vi "SVXMPL_Initialize.vi"(0 "device":i16=1, 1 "acquisition type":T1(ring), 5 "output channels":tag[](array[tag]), 9 "input channels":tag[](array[tag]), 11 "error in (no error)":errorcluster) -> (4 "acquisition task":T2={"AI device settings"={"AI device"=1, "AI taskID"=0, "response"=[]}, "acquisition type"=enum."Finite", "measurement settings"={"AI sampling frequency"=51200.0, "AO sampling frequency"=51200.0, "AI block size"=1024, "AO block Size"=0, "block duration [ms]"=1024.0, "number of AI channels"=0, "board propagation time [samples]"=0, "DUT propagation time [s]"=0.0}, "settling settings"={"settle time"=0.015599999576807022, "settle cycles"=5}, "integration settings"={"integration time"=0.015599999576807022, "integration cycles"=5}, "AO device settings"={"AO device"=1, "AO taskID"=0, "excitation"=[]}, "acquisition accounting"={"initial read size [samples]"=0, "read offset [samples]"=0, "read length [samples]"=0, "blocks to settle [samples]"=0, "min delay until transition [samples]"=0}, "frequency range"={"start frequency"=0.015599999576807022, "stop frequency"=5.0}, "block type"=enum."Initialize", "source settings"={"signal type"=enum."Dual tone (IMD)", "frequency"=0.0, "total amplitude"=0.0, "frequencies"=[1.0], "relative amplitudes"=[1.0], "offset"=1.0, "total amplitude list"=[1.0], "ramping rate"=0.0}} {"source settings"."total amplitude" format="%.2f"; "source settings"."relative amplitudes" format="%.2f"; "source settings"."frequencies" format="%.2f"; "source settings"."total amplitude list" format="%.2f"; "source settings"."ramping rate" format="%.4f"; "source settings"."offset" format="%.2f"; "source settings"."frequency" format="%.2f"; "frequency range"."stop frequency" format="%.2f"; "frequency range"."start frequency" format="%.2f"; "AO device settings"."excitation"."output limits"."low limit (-10 V)" format="%.2f"; "AO device settings"."excitation"."output limits"."high limit (10 V)" format="%.2f"; "AI device settings"."response"."input limits"."low limit (0.0)" format="%.2f"; "AI device settings"."response"."input limits"."high limit (0.0)" format="%.2f"; "integration settings"."integration time" format="%.2p"; "settling settings"."settle time" format="%.2p"; "measurement settings"."DUT propagation time [s]" format="%.2f"; "measurement settings"."AO sampling frequency" format="%.2f"; "measurement settings"."AI sampling frequency" format="%.2f"}, 15 "error out":errorcluster)   [LabVIEW 2017]
doc: "This example VI allows you to configure the <B>device</B>, <B>output channel</B>, and <B>input channels</B> that will be used for the synchronized AO/AI measurement. The device must support both input and output to use this VI.\n\nYou must also specify the <B>aquisition type</B> that will be performed.\n\"Finite\" is a one-shot measurement.\n\"Averaged\" is a continuous measurement in which measured blocks are averaged.\n\"Settled\" is a continuous measurement in which measured blocks are tested against the settling criteria. If the measurement is settled, only the last measurement is returned.\n\"Amplitude sweep\" is a continuous measurement in which each measured block has a different amplitude for the test signal."
uses:
  <vilib>/addons/Sound and Vibration/compatibility/Example Support/SVXMPL_Acquisition Task.ctl
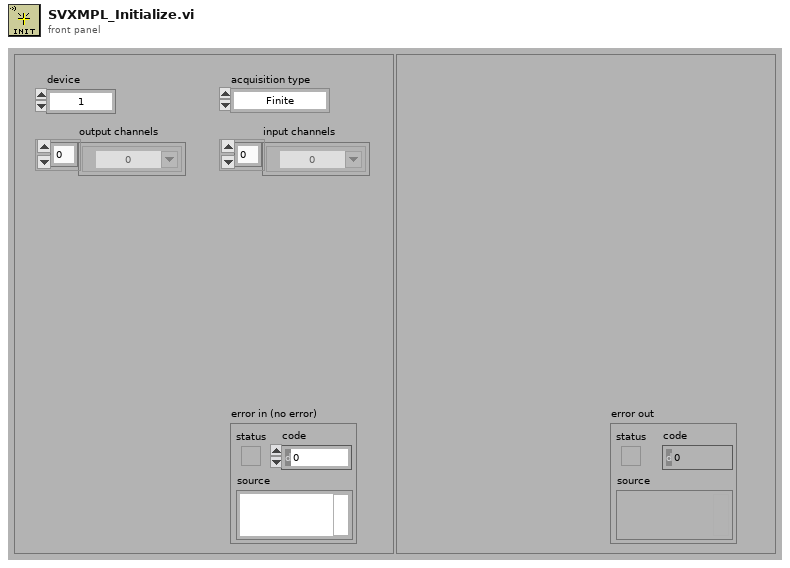
[diagram p1: front panel]
types:
  T1 = enum16{"Finite", "Averaged", "Settled", "Amplitude Sweep"}
  T2 = typedef "SVXMPL_Acquisition Task.ctl" = cluster{"AI device settings":cluster{"AI device":i16, "AI taskID":u32, "response":cluster{"AI channel":tag, "input limits":cluster{"high limit (0.0)":sgl, "low limit (0.0)":sgl}, "coupling & input config":cluster{"coupling":enum16{"no change", "DC", "AC", "GND", "internal ref."}, "input config":enum16{"no change", "differential", "ref. single-ended", "non-ref. single-ended", "4-wire"}}}[]}, "acquisition type":enum16{"Finite", "Averaged", "Settled", "Amplitude Sweep"}, "measurement settings":cluster{"AI sampling frequency":dbl, "AO sampling frequency":dbl, "AI block size":i32, "AO block Size":i32, "block duration [ms]":dbl, "number of AI channels":i32, "board propagation time [samples]":i32, "DUT propagation time [s]":dbl}, "settling settings":cluster{"settle time":dbl, "settle cycles":i32}, "integration settings":cluster{"integration time":dbl, "integration cycles":i32}, "AO device settings":cluster{"AO device":i16, "AO taskID":u32, "excitation":cluster{"AO Channel":tag, "output limits":cluster{"high limit (10 V)":sgl, "low limit (-10 V)":sgl, "reference source":enum16{"no change", "internal", "external"}}}[]}, "acquisition accounting":cluster{"initial read size [samples]":i32, "read offset [samples]":i32, "read length [samples]":i32, "blocks to settle [samples]":i32, "min delay until transition [samples]":i32}, "frequency range":cluster{"start frequency":dbl, "stop frequency":dbl}, "block type":enum16{"Initialize", "Settle", "Integrate"}, "source settings":cluster{"signal type":enum16{"Sine wave", "Dual tone (IMD)", "Multitone", "Chirp", "Frequency flat chirp", "Uniform white noise", "Gaussian white noise", "Pink noise", "PRN"}, "frequency":dbl, "total amplitude":dbl, "frequencies":dbl[], "relative amplitudes":dbl[], "offset":dbl, "total amplitude list":dbl[], "ramping rate":dbl}}
  T3 = cluster{"high limit (10 V)":sgl, "low limit (-10 V)":sgl, "reference source":enum16{"no change", "internal", "external"}}
  T4 = cluster{"coupling":enum16{"no change", "DC", "AC", "GND", "internal ref."}, "input config":enum16{"no change", "differential", "ref. single-ended", "non-ref. single-ended", "4-wire"}}
  T5 = cluster{"high limit (0.0)":sgl, "low limit (0.0)":sgl}
  T6 = cluster{"output channel":tag, "output limits":cluster{"high limit (10 V)":sgl, "low limit (-10 V)":sgl, "reference source":enum16{"no change", "internal", "external"}}}
  T7 = cluster{"input channel":tag, "input limits":cluster{"high limit (0.0)":sgl, "low limit (0.0)":sgl}, "coupling & input config":cluster{"coupling":enum16{"no change", "DC", "AC", "GND", "internal ref."}, "input config":enum16{"no change", "differential", "ref. single-ended", "non-ref. single-ended", "4-wire"}}}
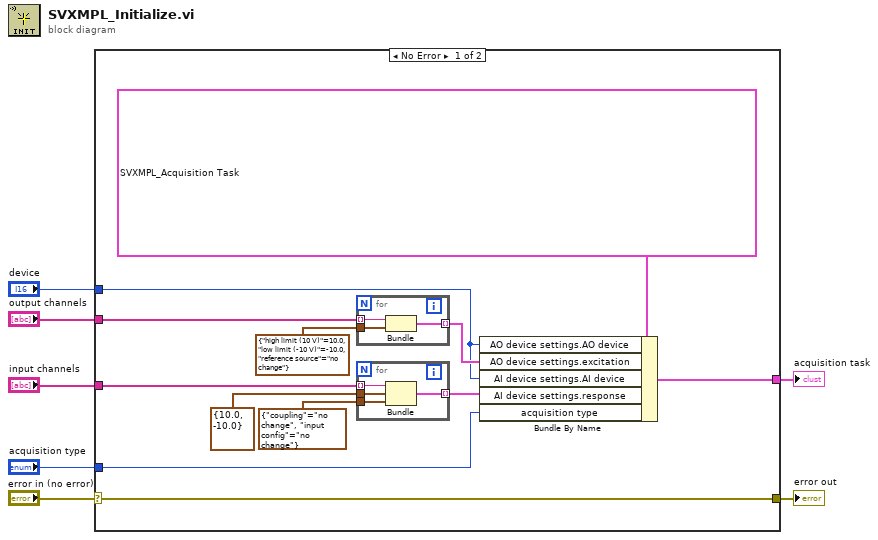
[diagram p0: block diagram]
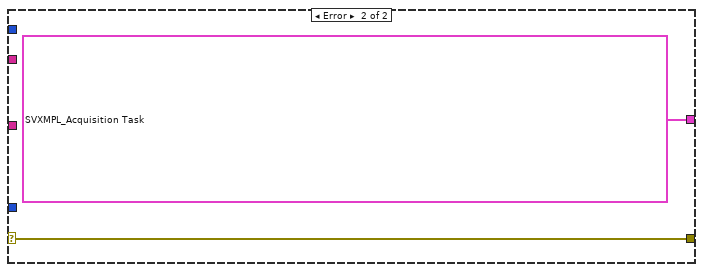
[diagram p2: hidden frame]
diagram:
  n1 = case shown="No Error" "error in (no error)" {
    selector: "error in (no error)" -> [w8 w27]
    tunnel: [w18 T2 {"AI device settings"={"AI device"=0, "AI taskID"=0, "response"=[{"AI channel"="0", "input limits"={"high limit (0.0)"=nan, "low limit (0.0)"=nan}, "coupling & input config"={"coupling"=enum."no change", "input config"=enum."no change"}}]}, "acquisition type"=enum."Finite", "measurement settings"={"AI sampling frequency"=nan, "AO sampling frequency"=nan, "AI block size"=0, "AO block Size"=0, "block duration [ms]"=nan, "number of AI channels"=0, "board propagation time [samples]"=0, "DUT propagation time [s]"=0.0}, "settling settings"={"settle time"=0.015599999576807022, "settle cycles"=5}, "integration settings"={"integration time"=0.015599999576807022, "integration cycles"=5}, "AO device settings"={"AO device"=1, "AO taskID"=0, "excitation"=[]}, "acquisition accounting"={"initial read size [samples]"=0, "read offset [samples]"=0, "read length [samples]"=0, "blocks to settle [samples]"=0, "min delay until transition [samples]"=0}, "frequency range"={"start frequency"=nan, "stop frequency"=0.0}, "block type"=enum."Initialize", "source settings"={"signal type"=enum."Sine wave", "frequency"=0.0, "total amplitude"=1.0, "frequencies"=[1.0], "relative amplitudes"=[1.0], "offset"=1.0, "total amplitude list"=[1.0], "ramping rate"=0.0}} ("acquisition task")] -> w7
    tunnel: "input channels" -> [w16 _]
    tunnel: "output channels" -> [w14 _]
    tunnel: "device" -> [w11 _]
    tunnel: "acquisition type" -> [w10 _]
    tunnel: [w8 w27] -> w1
    frame No Error {
      n2 = for {
        tunnel: w14 -> [w22] mode=indexing
        tunnel: T3 {"high limit (10 V)"=10.0, "low limit (-10 V)"=-10.0, "reference source"=enum."no change"} ("output limits") -> [w21]
        tunnel: [w20] -> w13 mode=indexing
        n3 = Bundle("output channel"=w22, "output limits"=w21) -> (w20:T6)  [unwired: 1 in]
      }
      n4 = for {
        tunnel: w16 -> [w26] mode=indexing
        tunnel: T5 {"high limit (0.0)"=10.0, "low limit (0.0)"=-10.0} ("input limits") -> [w25]
        tunnel: T4 {"coupling"=enum."no change", "input config"=enum."no change"} ("coupling & input config") -> [w24]
        tunnel: [w23] -> w15 mode=indexing
        n5 = Bundle("input channel"=w26, "input limits"=w25, "coupling & input config"=w24) -> (w23:T7)  [unwired: 1 in]
      }
      n6 = Bundle By Name(cluster=T2 {"AI device settings"={"AI device"=-1, "AI taskID"=0, "response"=[{"AI channel"="-0", "input limits"={"high limit (0.0)"=-1.0, "low limit (0.0)"=-1.0}, "coupling & input config"={"coupling"=enum."no change", "input config"=enum."no change"}}]}, "acquisition type"=enum."Finite", "measurement settings"={"AI sampling frequency"=0.0, "AO sampling frequency"=0.0, "AI block size"=0, "AO block Size"=0, "block duration [ms]"=0.0, "number of AI channels"=0, "board propagation time [samples]"=0, "DUT propagation time [s]"=0.0}, "settling settings"={"settle time"=0.015599999576807022, "settle cycles"=5}, "integration settings"={"integration time"=0.015599999576807022, "integration cycles"=5}, "AO device settings"={"AO device"=1, "AO taskID"=0, "excitation"=[]}, "acquisition accounting"={"initial read size [samples]"=0, "read offset [samples]"=0, "read length [samples]"=0, "blocks to settle [samples]"=0, "min delay until transition [samples]"=0}, "frequency range"={"start frequency"=0.0, "stop frequency"=0.0}, "block type"=enum."Initialize", "source settings"={"signal type"=enum."Sine wave", "frequency"=0.0, "total amplitude"=1.0, "frequencies"=[1.0], "relative amplitudes"=[1.0], "offset"=1.0, "total amplitude list"=[1.0], "ramping rate"=0.0}} ("acquisition task"), "AO device settings.AO device"=w11, "AO device settings.excitation"=w13, "AI device settings.AI device"=w11, "AI device settings.response"=w15, "acquisition type"=w10) -> (w18:T2)
    }
    frame Error {
    }
  }
  "acquisition task" <- w7
  "error out" <- w1
